vi "CRYUnflatten ViewProperty.vi"(11 "Flatten ViewPro":string) -> (0 "Error?":bool=TRUE, 2 "ViewPro Cluster":T1[](array[typedef]), 3 "Header info":T2={"Data type"="Data            ", "Version"=1, "Dimensions"=0})   [LabVIEW 2013]
uses:
  Control/CRYGraph Property.ctl
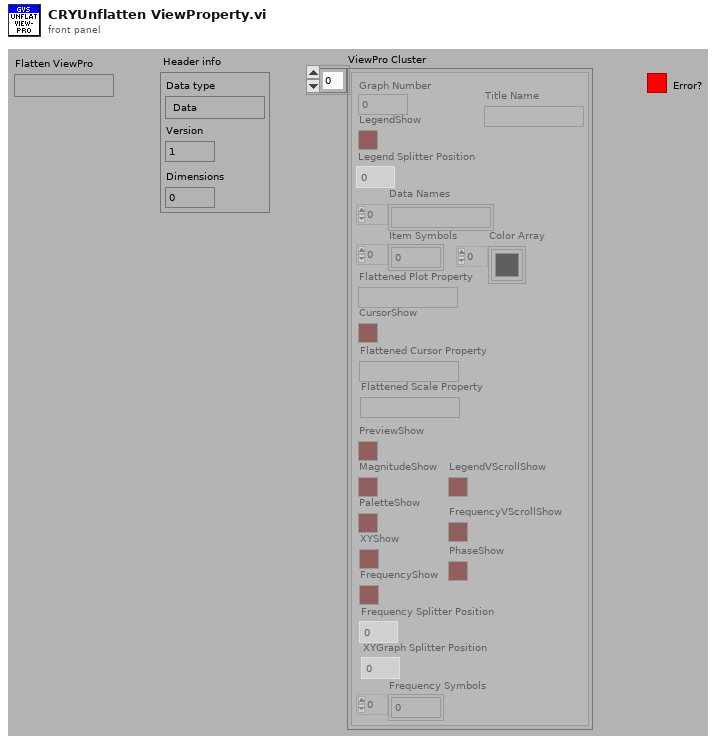
[diagram p1: front panel]
types:
  T1 = typedef "CRYGraph Property.ctl" = cluster{"LegendShow":bool, "Legend Splitter Position":dbl, "Data Names":string[], "Item Symbols":i32[], "Color Array":u32[], "Flattened Plot Property":string, "CursorShow":bool, "Flattened Cursor Property":string, "Graph Number":i32, "Flattened Scale Property":string, "PreviewShow":bool, "MagnitudeShow":bool, "PaletteShow":bool, "XYShow":bool, "FrequencyShow":bool, "Frequency Splitter Position":dbl, "XYGraph Splitter Position":dbl, "Frequency Symbols":i32[], "LegendVScrollShow":bool, "FrequencyVScrollShow":bool, "PhaseShow":bool, "Title Name":string}
  T2 = cluster{"Data type":string, "Version":u16, "Dimensions":u8}
  T3 = cluster{"unsigned byte array[0]":u8, "unsigned byte array[1]":u8, "unsigned byte array[2]":u8}
  T4 = cluster{"LegendShow":bool, "Legend Splitter Position":dbl, "Data Names":string[], "Item Symbols":i32[], "Color Array":u32[], "Flattened Plot Property":string, "CursorShow":bool, "Flattened Cursor Property":string, "Graph Number":i32, "Flattened Scale Property":string}[]
  T5 = cluster{"LegendShow":bool, "Legend Splitter Position":dbl, "Data Names":string[], "Item Symbols":i32[], "Color Array":u32[], "Flattened Plot Property":string, "CursorShow":bool, "Flattened Cursor Property":string, "Graph Number":i32, "Flattened Scale Property":string, "PreviewShow":bool, "MagnitudeShow":bool, "PaletteShow":bool}[]
  T6 = cluster{"LegendShow":bool, "Legend Splitter Position":dbl, "Data Names":string[], "Item Symbols":i32[], "Color Array":u32[], "Flattened Plot Property":string, "CursorShow":bool, "Flattened Cursor Property":string, "Graph Number":i32, "Flattened Scale Property":string, "PreviewShow":bool, "MagnitudeShow":bool, "PaletteShow":bool, "XYShow":bool, "FrequencyShow":bool, "Frequency Splitter Position":dbl, "XYGraph Splitter Position":dbl, "Frequency Symbols":i32[]}[]
  T7 = cluster{"LegendShow":bool, "Legend Splitter Position":dbl, "Data Names":string[], "Item Symbols":i32[], "Color Array":u32[], "Flattened Plot Property":string, "CursorShow":bool, "Flattened Cursor Property":string, "Graph Number":i32, "Flattened Scale Property":string, "PreviewShow":bool, "MagnitudeShow":bool, "PaletteShow":bool, "XYShow":bool, "FrequencyShow":bool, "Frequency Splitter Position":dbl, "XYGraph Splitter Position":dbl, "Frequency Symbols":i32[], "LegendVScrollShow":bool}[]
  T8 = cluster{"LegendShow":bool, "Legend Splitter Position":dbl, "Data Names":string[], "Item Symbols":i32[], "Color Array":u32[], "Flattened Plot Property":string, "CursorShow":bool, "Flattened Cursor Property":string, "Graph Number":i32, "Flattened Scale Property":string, "PreviewShow":bool, "MagnitudeShow":bool, "PaletteShow":bool, "XYShow":bool, "FrequencyShow":bool, "Frequency Splitter Position":dbl, "XYGraph Splitter Position":dbl, "Frequency Symbols":i32[], "LegendVScrollShow":bool, "FrequencyVScrollShow":bool}[]
  T9 = cluster{"substring":string, u16, "unsigned byte array[2]":u8}
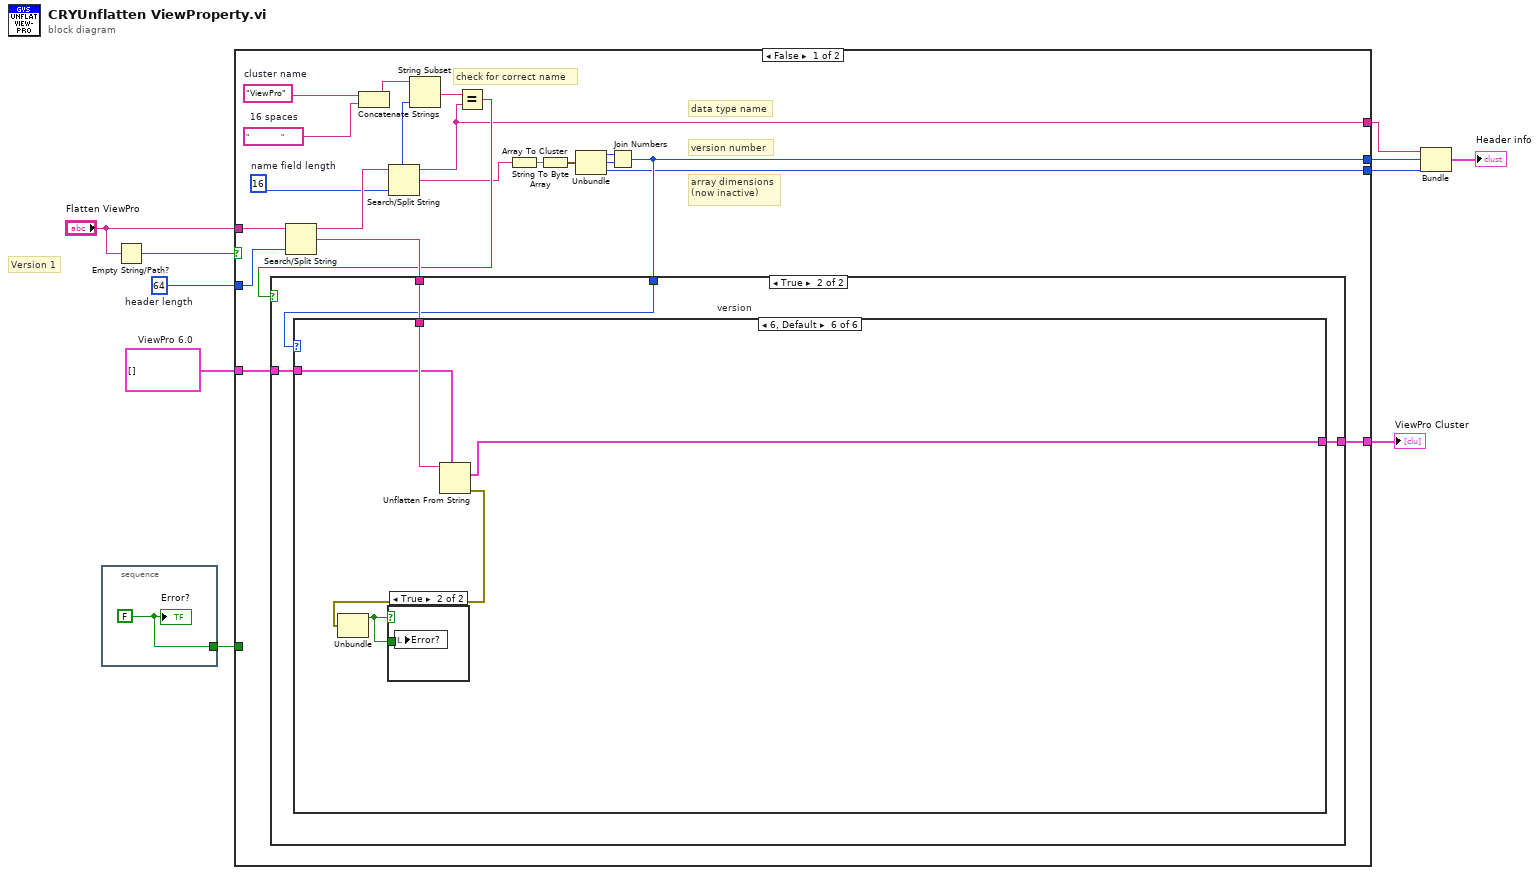
[diagram p0: block diagram]
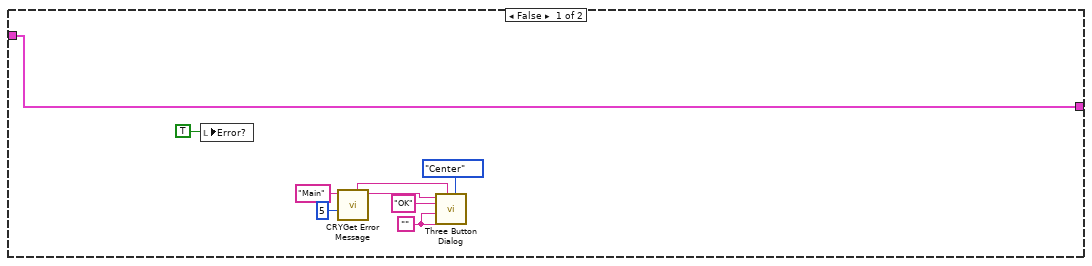
[diagram p2: hidden frame]
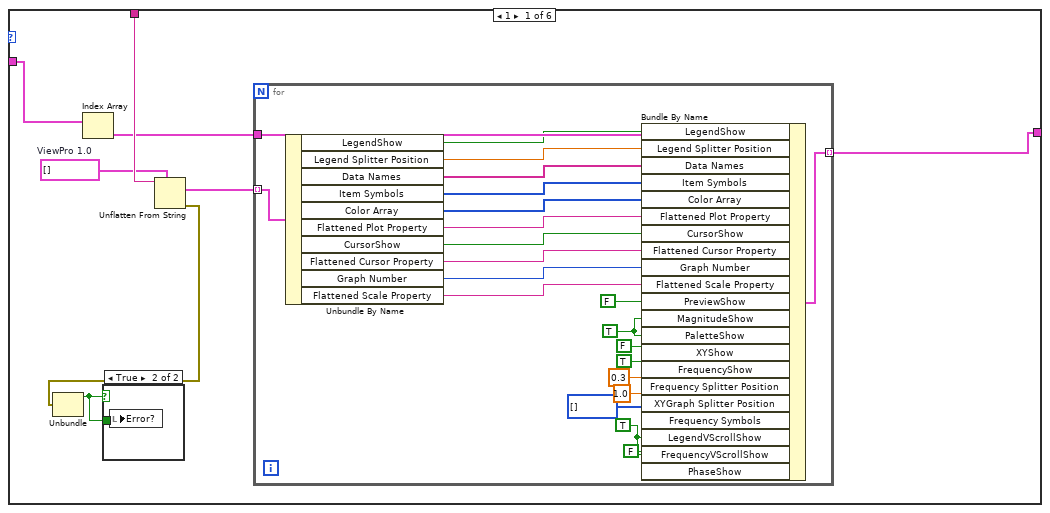
[diagram p3: hidden frame]
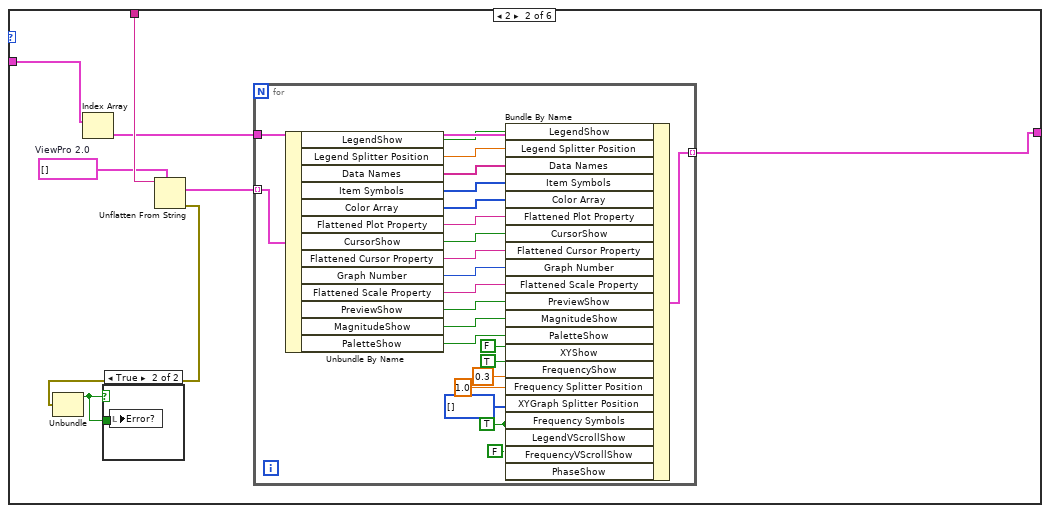
[diagram p5: hidden frame]
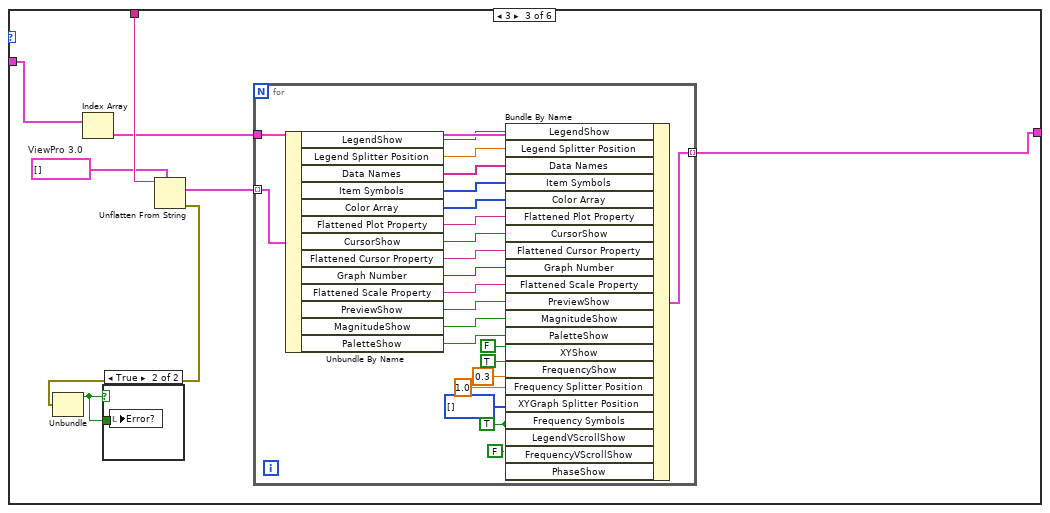
[diagram p7: hidden frame]
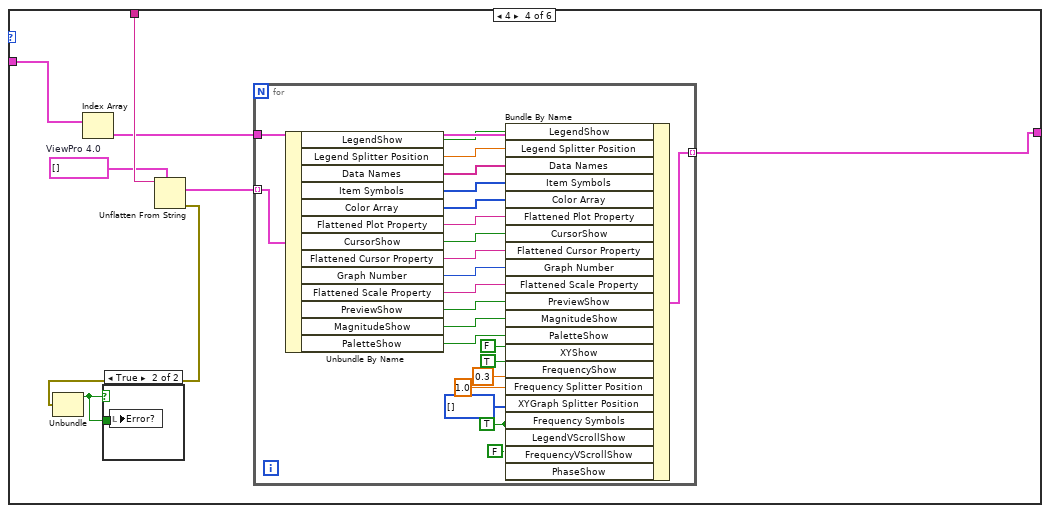
[diagram p9: hidden frame]
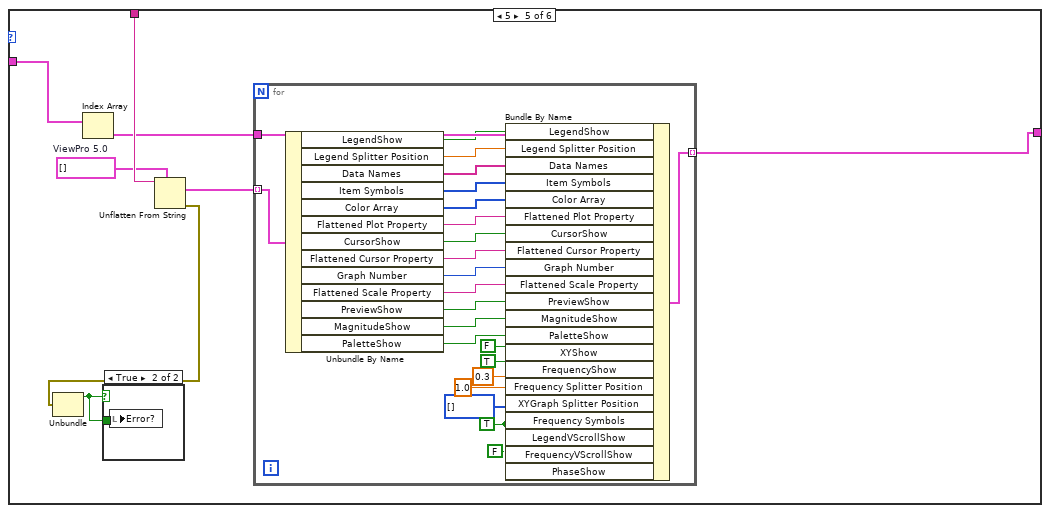
[diagram p11: hidden frame]
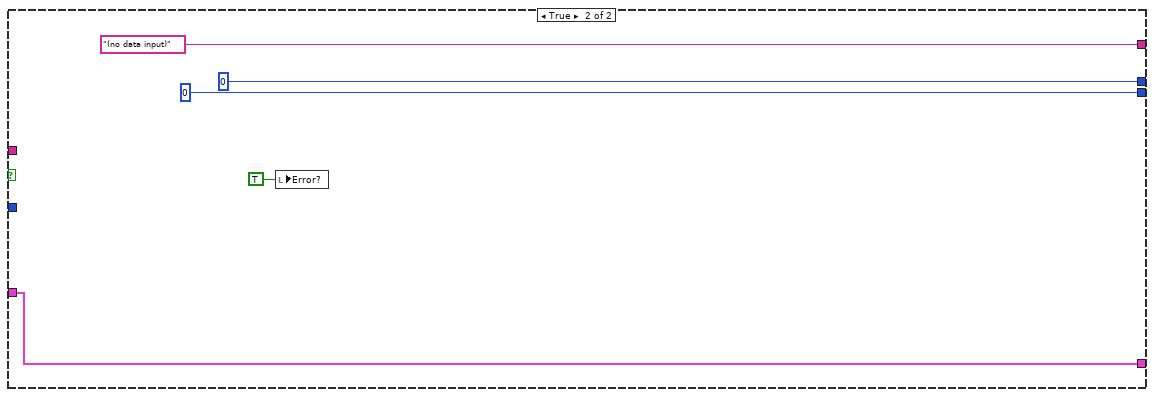
[diagram p14: hidden frame]
diagram:
  w2 = T1[] []  # ViewPro 6.0
  w8 = 64  # header length
  # "Version 1"
  n1 = stacked-sequence {
    tunnel: [w11] -> w3
    frame #0 {
      w11 = FALSE
      "Error?" <- w11
    }
  }
  n2 = Empty String/Path?(string/path="Flatten ViewPro") -> (empty?=w9:bool)
  n3 = case shown="False" w9 {
    tunnel: "Flatten ViewPro" -> [w31 _]
    tunnel: w8 -> [w25 _]
    tunnel: [w22 u16 0] -> w6
    tunnel: [w14 u8 0] -> w7
    tunnel: [w15 "(no data input)" ("substring")] -> w5
    tunnel: w3 -> [_ _]
    tunnel: [w13 w210] -> w1
    tunnel: w2 -> [w12 w210]
    frame False {
      w19 = "                "  # 16 spaces
      w20 = "ViewPro"  # cluster name
      w17 = 16  # name field length
      # "check for correct name"
      # "array dimensions\n(now inactive)"
      # "version number"
      # "data type name"
      n4 = Search/Split String(string=w31, offset (0)=w25) -> (substring before match=w24:string, match + rest of string=w26:string)  [unwired: 2 out]
      n5 = Concatenate Strings(w20, w19) -> (w18:string)
      n6 = Search/Split String(string=w24, offset (0)=w17) -> (substring before match=w15:string, match + rest of string=w21:string)  [unwired: 2 out]
      n7 = String Subset(string=w18, length (rest)=w17) -> (substring=w16:string)  [unwired: 1 out]
      n8 = Equal?(x=w16, y=w15) -> (x = y?=w23:bool)
      n9 = String To Byte Array(string=w21) -> (unsigned byte array=w30:u8[])
      n10 = Array To Cluster(array=w30) -> (cluster=w29:T3)
      n11 = Unbundle(w29) -> ("unsigned byte array[0]"=w28:u8, "unsigned byte array[1]"=w27:u8, "unsigned byte array[2]"=w14:u8)
      n12 = Join Numbers(hi=w28, lo=w27) -> ((hi.lo)=w22:u16)
      n13 = case shown="True" w23 {
        tunnel: w26 -> [_ w44]
        tunnel: w22 -> [_ w43]
        tunnel: [w32 w42] -> w13
        tunnel: w12 -> [w32 w41]
        frame False {
          w39 = ""
          n14 = local write "Error?"(TRUE) -> ()
          n15 = call "CRYGet Error Message.vi"("Error No"=5, "Kind"="Main") -> ("Message"=w34:string, "Window Title"=w33:string)  [unwired: 4 in, 4 out]
          n16 = call <vilib>:"Three Button Dialog.vi"("Justify Message (Left)"=enum16{"Left", "Center", "Right"}."Center", "Window Title (\"\")"=w33, "Right Button Text (\"Cancel\")"=w39, "Center Button Text (\"No\")"=w39, "Left Button Text (\"Yes\")"="OK" ("Left Button Text (\"Yes\")"), "message"=w34) -> ()  [unwired: 6 out]
        }
        frame True {
          n17 = case "version" shown="6, Default" w43 {
            tunnel: w44 -> [w52 w83 w115 w147 w179 w208]
            tunnel: [w47 w78 w110 w142 w174 w205] -> w42
            tunnel: w41 -> [w46 w77 w109 w141 w173 w204]
            frame 1 {
              w45 = T4 []  # ViewPro 1.0
              n18 = Index Array(array=w46) -> (element=w49:T1)  [unwired: 1 in]
              n19 = Unflatten From String(type=w45, binary string=w52) -> (value=w48:T4, error out=w50:errorcluster)  [unwired: 1 in, 3 out]
              n20 = Unbundle(w50) -> ("status"=w51:bool)  [unwired: 2 out]
              n21 = case shown="True" w51 {
                tunnel: w51 -> [_ w75]
                frame False {
                }
                frame True {
                  n22 = local write "Error?"(w75) -> ()
                }
              }
              n23 = for {
                tunnel: w49 -> [w73]
                tunnel: w48 -> [w74] mode=indexing
                tunnel: [w72] -> w47 mode=indexing
                w54 = TRUE ("LegendVScrollShow")
                w61 = TRUE ("PaletteShow")
                n24 = Unbundle By Name(w74) -> ("LegendShow"=w71:bool, "Legend Splitter Position"=w70:dbl, "Data Names"=w56:string[], "Item Symbols"=w69:i32[], "Color Array"=w68:u32[], "Flattened Plot Property"=w67:string, "CursorShow"=w66:bool, "Flattened Cursor Property"=w65:string, "Graph Number"=w64:i32, "Flattened Scale Property"=w63:string)
                n25 = Bundle By Name(cluster=w73, "LegendShow"=w71, "Legend Splitter Position"=w70, "Data Names"=w56, "Item Symbols"=w69, "Color Array"=w68, "Flattened Plot Property"=w67, "CursorShow"=w66, "Flattened Cursor Property"=w65, "Graph Number"=w64, "Flattened Scale Property"=w63, "PreviewShow"=FALSE, "MagnitudeShow"=w61, "PaletteShow"=w61, "XYShow"=FALSE, "FrequencyShow"=TRUE, "Frequency Splitter Position"=0.3, "XYGraph Splitter Position"=1.0, "Frequency Symbols"=i32[] [], "LegendVScrollShow"=w54, "FrequencyVScrollShow"=w54, "PhaseShow"=FALSE) -> (w72:T1)
              }
            }
            frame 2 {
              w76 = T5 []  # ViewPro 2.0
              n26 = Index Array(array=w77) -> (element=w80:T1)  [unwired: 1 in]
              n27 = Unflatten From String(type=w76, binary string=w83) -> (value=w79:T5, error out=w81:errorcluster)  [unwired: 1 in, 3 out]
              n28 = Unbundle(w81) -> ("status"=w82:bool)  [unwired: 2 out]
              n29 = case shown="True" w82 {
                tunnel: w82 -> [_ w107]
                frame False {
                }
                frame True {
                  n30 = local write "Error?"(w107) -> ()
                }
              }
              n31 = for {
                tunnel: w80 -> [w105]
                tunnel: w79 -> [w106] mode=indexing
                tunnel: [w104] -> w78 mode=indexing
                w85 = TRUE ("LegendVScrollShow")
                n32 = Unbundle By Name(w106) -> ("LegendShow"=w103:bool, "Legend Splitter Position"=w102:dbl, "Data Names"=w101:string[], "Item Symbols"=w100:i32[], "Color Array"=w99:u32[], "Flattened Plot Property"=w98:string, "CursorShow"=w97:bool, "Flattened Cursor Property"=w96:string, "Graph Number"=w95:i32, "Flattened Scale Property"=w94:string, "PreviewShow"=w93:bool, "MagnitudeShow"=w92:bool, "PaletteShow"=w91:bool)
                n33 = Bundle By Name(cluster=w105, "LegendShow"=w103, "Legend Splitter Position"=w102, "Data Names"=w101, "Item Symbols"=w100, "Color Array"=w99, "Flattened Plot Property"=w98, "CursorShow"=w97, "Flattened Cursor Property"=w96, "Graph Number"=w95, "Flattened Scale Property"=w94, "PreviewShow"=w93, "MagnitudeShow"=w92, "PaletteShow"=w91, "XYShow"=FALSE, "FrequencyShow"=TRUE, "Frequency Splitter Position"=0.3, "XYGraph Splitter Position"=1.0, "Frequency Symbols"=i32[] [], "LegendVScrollShow"=w85, "FrequencyVScrollShow"=w85, "PhaseShow"=FALSE) -> (w104:T1)
              }
            }
            frame 3 {
              w108 = T6 []  # ViewPro 3.0
              n34 = Index Array(array=w109) -> (element=w112:T1)  [unwired: 1 in]
              n35 = Unflatten From String(type=w108, binary string=w115) -> (value=w111:T6, error out=w113:errorcluster)  [unwired: 1 in, 3 out]
              n36 = Unbundle(w113) -> ("status"=w114:bool)  [unwired: 2 out]
              n37 = case shown="True" w114 {
                tunnel: w114 -> [_ w139]
                frame False {
                }
                frame True {
                  n38 = local write "Error?"(w139) -> ()
                }
              }
              n39 = for {
                tunnel: w112 -> [w137]
                tunnel: w111 -> [w138] mode=indexing
                tunnel: [w136] -> w110 mode=indexing
                w117 = TRUE ("LegendVScrollShow")
                n40 = Unbundle By Name(w138) -> ("LegendShow"=w135:bool, "Legend Splitter Position"=w134:dbl, "Data Names"=w133:string[], "Item Symbols"=w132:i32[], "Color Array"=w131:u32[], "Flattened Plot Property"=w130:string, "CursorShow"=w129:bool, "Flattened Cursor Property"=w128:string, "Graph Number"=w127:i32, "Flattened Scale Property"=w126:string, "PreviewShow"=w125:bool, "MagnitudeShow"=w124:bool, "PaletteShow"=w123:bool)
                n41 = Bundle By Name(cluster=w137, "LegendShow"=w135, "Legend Splitter Position"=w134, "Data Names"=w133, "Item Symbols"=w132, "Color Array"=w131, "Flattened Plot Property"=w130, "CursorShow"=w129, "Flattened Cursor Property"=w128, "Graph Number"=w127, "Flattened Scale Property"=w126, "PreviewShow"=w125, "MagnitudeShow"=w124, "PaletteShow"=w123, "XYShow"=FALSE, "FrequencyShow"=TRUE, "Frequency Splitter Position"=0.3, "XYGraph Splitter Position"=1.0, "Frequency Symbols"=i32[] [], "LegendVScrollShow"=w117, "FrequencyVScrollShow"=w117, "PhaseShow"=FALSE) -> (w136:T1)
              }
            }
            frame 4 {
              w140 = T7 []  # ViewPro 4.0
              n42 = Index Array(array=w141) -> (element=w144:T1)  [unwired: 1 in]
              n43 = Unflatten From String(type=w140, binary string=w147) -> (value=w143:T7, error out=w145:errorcluster)  [unwired: 1 in, 3 out]
              n44 = Unbundle(w145) -> ("status"=w146:bool)  [unwired: 2 out]
              n45 = case shown="True" w146 {
                tunnel: w146 -> [_ w171]
                frame False {
                }
                frame True {
                  n46 = local write "Error?"(w171) -> ()
                }
              }
              n47 = for {
                tunnel: w144 -> [w169]
                tunnel: w143 -> [w170] mode=indexing
                tunnel: [w168] -> w142 mode=indexing
                w149 = TRUE ("LegendVScrollShow")
                n48 = Unbundle By Name(w170) -> ("LegendShow"=w167:bool, "Legend Splitter Position"=w166:dbl, "Data Names"=w165:string[], "Item Symbols"=w164:i32[], "Color Array"=w163:u32[], "Flattened Plot Property"=w162:string, "CursorShow"=w161:bool, "Flattened Cursor Property"=w160:string, "Graph Number"=w159:i32, "Flattened Scale Property"=w158:string, "PreviewShow"=w157:bool, "MagnitudeShow"=w156:bool, "PaletteShow"=w155:bool)
                n49 = Bundle By Name(cluster=w169, "LegendShow"=w167, "Legend Splitter Position"=w166, "Data Names"=w165, "Item Symbols"=w164, "Color Array"=w163, "Flattened Plot Property"=w162, "CursorShow"=w161, "Flattened Cursor Property"=w160, "Graph Number"=w159, "Flattened Scale Property"=w158, "PreviewShow"=w157, "MagnitudeShow"=w156, "PaletteShow"=w155, "XYShow"=FALSE, "FrequencyShow"=TRUE, "Frequency Splitter Position"=0.3, "XYGraph Splitter Position"=1.0, "Frequency Symbols"=i32[] [], "LegendVScrollShow"=w149, "FrequencyVScrollShow"=w149, "PhaseShow"=FALSE) -> (w168:T1)
              }
            }
            frame 5 {
              w172 = T8 []  # ViewPro 5.0
              n50 = Index Array(array=w173) -> (element=w176:T1)  [unwired: 1 in]
              n51 = Unflatten From String(type=w172, binary string=w179) -> (value=w175:T8, error out=w177:errorcluster)  [unwired: 1 in, 3 out]
              n52 = Unbundle(w177) -> ("status"=w178:bool)  [unwired: 2 out]
              n53 = case shown="True" w178 {
                tunnel: w178 -> [_ w203]
                frame False {
                }
                frame True {
                  n54 = local write "Error?"(w203) -> ()
                }
              }
              n55 = for {
                tunnel: w176 -> [w201]
                tunnel: w175 -> [w202] mode=indexing
                tunnel: [w200] -> w174 mode=indexing
                w181 = TRUE ("LegendVScrollShow")
                n56 = Unbundle By Name(w202) -> ("LegendShow"=w199:bool, "Legend Splitter Position"=w198:dbl, "Data Names"=w197:string[], "Item Symbols"=w196:i32[], "Color Array"=w195:u32[], "Flattened Plot Property"=w194:string, "CursorShow"=w193:bool, "Flattened Cursor Property"=w192:string, "Graph Number"=w191:i32, "Flattened Scale Property"=w190:string, "PreviewShow"=w189:bool, "MagnitudeShow"=w188:bool, "PaletteShow"=w187:bool)
                n57 = Bundle By Name(cluster=w201, "LegendShow"=w199, "Legend Splitter Position"=w198, "Data Names"=w197, "Item Symbols"=w196, "Color Array"=w195, "Flattened Plot Property"=w194, "CursorShow"=w193, "Flattened Cursor Property"=w192, "Graph Number"=w191, "Flattened Scale Property"=w190, "PreviewShow"=w189, "MagnitudeShow"=w188, "PaletteShow"=w187, "XYShow"=FALSE, "FrequencyShow"=TRUE, "Frequency Splitter Position"=0.3, "XYGraph Splitter Position"=1.0, "Frequency Symbols"=i32[] [], "LegendVScrollShow"=w181, "FrequencyVScrollShow"=w181, "PhaseShow"=FALSE) -> (w200:T1)
              }
            }
            frame 6, Default {
              n58 = Unflatten From String(type=w204, binary string=w208) -> (value=w205:T1[], error out=w206:errorcluster)  [unwired: 1 in, 3 out]
              n59 = Unbundle(w206) -> ("status"=w207:bool)  [unwired: 2 out]
              n60 = case shown="True" w207 {
                tunnel: w207 -> [_ w209]
                frame False {
                }
                frame True {
                  n61 = local write "Error?"(w209) -> ()
                }
              }
            }
          }
        }
      }
    }
    frame True {
      n62 = local write "Error?"(TRUE ("Error?")) -> ()
    }
  }
  "ViewPro Cluster" <- w1
  n63 = Bundle("substring"=w5, w6, "unsigned byte array[2]"=w7) -> (→"Header info":T9)  [unwired: 1 out]
